vi "App - analyze RUS V6.vi"() -> ()   [LabVIEW 2015] (continued)
  out "frequency points":dbl[](array[numeric])=[0.0, 0.0, 0.0, 0.0, 0.0, 0.0, 0.0, 0.0, 0.0, 0.0, 0.0, 0.0, 0.0, 0.0, 0.0, 0.0, 0.0, 0.0, 0.0, 0.0, 0.0, 0.0, 0.0, 0.0, 0.0, 0.0, 0.0, 0.0, 0.0, 0.0, 0.0, 0.0, 0.0, 0.0, 0.0, 0.0, 0.0, 0.0, 0.0, 0.0, 0.0, 0.0, 0.0, 0.0, 0.0, 0.0, 0.0, 0.0, 664.2436695290903, 664.2619309392137, 664.2805728990513, 664.2981443004336, 664.3188476258067, 664.3335964907527, 664.3536063641833, 664.3711441248129, 664.3886135894766, 664.4069577109009, 664.4245585272355, 664.4414683185125, 664.4601452577426, 664.4796852677678, 664.4980076667935, 664.5154310442224, 664.5338643964093, 664.5517885931691, 664.5704803534437, 664.588180324614, 664.6064246538435, 664.6239877084581, 664.6422601490035, 664.6602601074228, 664.6782562264044, 664.6963935252326, 664.7147754224831, 664.7329875150317, 664.7514539650158, 664.7696405311139, 664.7884789608521, 664.8081200534322, 664.8281506310057, 664.8464656256355, 664.8647360420077, 664.8826826665108, 664.9021630370361, 664.9200138534414, 664.9394190348338, 664.9570161356205, 664.9751037863994, 664.9946492766225, 665.013363493181, 665.0319666327775, 665.0514303799941, 665.070428839104, 665.0899681894765, 665.1092165846538, 665.128636002681, 665.1480453032892, 665.1669866582076, 665.185992115189, 665.2049981978538, 665.2252219651873, 665.2450117111404, 665.2636719185228, 665.2820790020305, 665.302621721353, 665.3209060628186, 665.3411726525135, 665.3602455630045, 665.3791825777425, 665.3983648536116, 665.4185749812924, 665.4389184365867, 665.4576110068883, 665.4746111668128, 665.4943966614766, 665.5130010905406, 665.532316198093, 665.5532332931765, 665.57156331953, 665.592509513559, 665.6111561314502, 665.6307876831706, 665.6495981705524, 665.6676827317286, 665.6875855513655, 665.7073536709393, 665.7270146903713, 665.7475776559688, 665.7667570785509, 665.7853656920117, 665.8055568664535, 665.8247976415821, 665.8450275889691, 665.8652215366186, 665.8855803249663, 665.9069182376624, 665.9269377443005, 665.9465552746622, 665.9681031960093, 665.9882719429886, 666.0103637387408, 666.0300130208008, 666.0483020662261, 666.067358184188, 666.0861004254415, 666.1047052834762, 666.12482136998, 666.140704057652, 666.1610854922133, 666.1802100253361, 666.2003193033272, 666.2201606193609, 666.23899502151, 666.257459442358, 666.2778888148354, 666.2970981562802, 666.3156869001568, 666.3357577270784, 666.3558831541329, 666.3762094650621, 666.3976643168794, 666.4187151485258, 666.4383021086978, 666.4551854285005, 666.4720190334131, 666.4896912216159, 666.5084730527226, 666.5273905158227, 666.5408565163474, 666.5638551761065, 666.584524931986, 666.5994517164672, 666.6209744644639, 666.6398754592545, 666.6584173096262, 666.6738278296584, 666.692959166971, 666.7084573649482, 666.7295180919369, 666.7478022514588, 666.7684075589387, 666.7892001669214, 666.8168017277993, 666.8378173116613, 666.8546119137043, 666.8518486216516, 666.8670899449811, 666.8864924413293, 666.9049225640731, 666.9154225888688, 666.9360592058572, 666.9893085918818, 667.023179450894, 667.0181290997397, 667.0522165263105, 667.0670953246381, 667.0830991408355, 667.0958987277553, 667.1178151875246, 667.1376282461717, 667.1555761001051, 667.1729816030107, 667.1877067469779, 667.2026820856647, 667.2204079387552, 667.2371268200717, 667.2364415496808, 667.2762898680271, 667.2972094216088, 667.3167356990505, 667.3324754640709, 667.3490257970444, 667.3649515647236, 667.3831987020516, 667.3988052282629, 667.4131682428546, 667.4308567999159, 667.4487531200956, 667.4658300241209, 667.4848884179092, 667.5023892207363, 667.5167865078748, 667.530667219577, 667.5446936387285, 667.5507361439306, 667.5713768371177, 667.5871571554018, 667.603372353538, 667.6196504795548, 667.6345004307237, 667.6414584582035, 667.6596980423662, 667.6762506062214, 667.6919916866713, 667.704330610667, 667.7178274337781, 667.7315679125422, 667.7469406174972, 667.7605274396784, 667.772514287168, 667.7857246989796, 667.7975632145829, 667.8113824108048, 667.8259629307869, 667.8339870162451, 667.846314585591, 667.8533606686503, 667.8697794122957, 667.8814288240087, 667.8943565204472, 667.9070637171257, 667.9189901657315, 667.9290708716037, 667.9412342117888, 667.9478689614617, 667.9595344300756, 667.9715429031386, 667.98053690319, 667.9933159378816, 668.0042574571033, 668.0186275854775, 668.0261021371313, 668.038205785295, 668.0502969770072, 668.0581032164006, 668.0629833326522, 668.0682070709669, 668.0806358264088, 668.0819765634108, 668.0941556665481, 668.1086689007784, 668.1154417247612, 668.1232509827006, 668.1252877234232, 668.1324581018087, 668.1449136803938, 668.1500479338042, 668.1552952835116, 668.1649667431813, 668.1727890439503, 668.1779102230967, 668.1880252548099, 668.192804963829, 668.2024272814265, 668.2077960895239, 668.216668111389, 668.2220891882298, 668.2279899714331, 668.2341074013727, 668.2403250081744, 668.2467222103966, 668.2497252249998, 668.2550593154574, 668.2609151074342, 668.2619254491482, 668.270115071191, 668.276245083583, 668.2795802722522, 668.2870233031718, 668.2869168107318, 668.2934784041765, 668.3008315870534, 668.3028814309054, 668.3062964998082, 668.3103990781085, 668.310674127471, 668.3160212015783, 668.3205621538442, 668.3261810591241, 668.3339307703254, 668.3324079597492, 668.3322615543187, 668.3288000801537, 668.3337947654519, 668.3393724178951, 668.3408415336296, 668.3350781624661, 668.341978511539, 668.3443633787955, 668.3397547361191, 668.338634717693, 668.3411059711797, 668.3387712789065, 668.3427557708224, 668.3438270287197, 668.3463481103089, 668.3455084349229, 668.3450708618282, 668.3433267141062, 668.3444873126522, 668.3461478794261, 668.3457969116931, 668.3464465453555, 668.3409387012916, 668.3392344820684, 668.3394447248988, 668.3369686011712, 668.3366293662327, 668.3323623372692, 668.3318352391343, 668.3346922322422, 668.3330864941908, 668.3219517274852, 668.3129997886653, 668.3140680165973, 668.3088794677242, 668.3109415026871, 668.3052156629583, 668.3064621156966, 668.2991530946135, 668.296337187602, 668.2941712628873, 668.2879323748828, 668.2827006729923, 668.2752935986506, 668.2706731525243, 668.265311084802, 668.2583083453824, 668.2568309954227, 668.251544958297, 668.2453085062731, 668.2394743021457, 668.2322266809226, 668.2226032955875, 668.2221912502285, 668.2178106776172, 668.2137975862624, 668.2079346540519, 668.2000760755379, 668.194062828963, 668.1891261636409, 668.1800061469135, 668.1744243080439, 668.167621356464, 668.1637736220466, 668.1572968562582, 668.1537550879266, 668.1449838049871, 668.135169475204, 668.1246913482574, 668.121193286822, 668.1101664128744, 668.0998885496297, 668.0911411970284, 668.0843412935199, 668.074848351984, 668.0672099835513, 668.0546726344026, 668.0432151630731, 668.0317886551247, 668.0206931728633, 668.0108019958866, 668.000884305955, 667.994986941211, 667.9845360403064, 667.9709114890906, 667.963154410693, 667.9559671880407, 667.9461007473978, 667.9364915226823, 667.9270848813279, 667.9206130476543, 667.9097751474013, 667.9032383407135, 667.900021351503, 667.8939948673919, 667.8857574673999, 667.8761489000353, 667.873197176711, 667.8687353967621, 667.8714445455947, 667.8742869887905, 667.8871818169091, 667.8929742135593, 667.8950769727215, 667.9087317249022, 667.9127020137031, 667.9290862382628, 667.9424835071507, 667.9529480751149, 667.9649600314765, 667.9769292525697, 667.9949531202576, 668.0129403654028, 668.0268805358065, 668.0419170256847, 668.0495978156077, 668.0649496135221, 668.0806226434124, 668.0882919601835, 668.0896160369514, 668.0963848127388, 668.0981322511478, 668.106726291208, 668.1148687330386, 668.1099013064036, 668.1117303235795, 668.1110147726321, 668.1116377961806, 668.1101255100197, 668.1053232498274, 668.1031913806788, 668.1004691432302, 668.0992433152304, 668.1003509236078, 668.1064053025405, 668.1052302227044, 668.1022726722371, 668.1004679566593, 668.0972424835554, 668.0965315443399, 668.0939847231178, 668.0907103744488, 668.0884812262261, 668.0853168502122, 668.0833849424677, 668.0812319431826, 668.076925264809, 668.0728404783213, 668.0649075247303, 668.0660057593828, 668.0603228410023, 668.0526848700105, 668.0459870419369, 668.0382438056512, 668.0317727144501, 668.0229320244955, 668.0104558389754, 668.0013835956787, 667.9844280868045, 667.9730328624377, 667.9597690228534, 667.9520044016398, 667.9421204350114, 667.9314512587483, 667.9245739426502, 667.915672183135, 667.9042185316268, 667.8931568087993, 667.8785430669695, 667.867203293899, 667.8547807071961, 667.8418460648647, 667.8284078259741, 667.8174456972619, 667.8098934060879, 667.7999931838958, 667.7879029943412, 667.7767811952523, 667.766686685923, 667.7537699797824, 667.7441411520185, 667.7346507175026, 667.7218411788447, 667.7090832290504, 667.6987650095127, 667.6847550615028, 667.6716677581467, 667.6622092104991, 667.6494194591486, 667.6370796373111, 667.6271523663532, 667.616063077065, 667.5996159742031, 667.5849862740106, 667.5706432660058, 667.555832927336, 667.5428492141318, 667.5298004796668, 667.515440025869, 667.4995586436626, 667.4860922618307, 667.4736345533211, 667.4573357267553, 667.4424028954636, 667.4251980802276, 667.41000498982, 667.3944561053353, 667.3780759125216, 667.3663738953067, 667.3507898349178, 667.3338926093543, 667.3173685004768, 667.3005746288229, 667.2855690828252, 667.2692762902061, 667.2515590922309, 667.231376618077, 667.2146515753702, 667.1959425135124, 667.1780248365252, 667.1610973636662, 667.1361303785343, 667.1181117945565, 667.0987327287644, 667.0822028525415, 667.0647376572853, 667.0441866711889, 667.0271022203252, 667.0058178404381, 666.9844113515632, 666.9627164169844, 666.9433323926924, 666.9265821241922, 666.9065573278365, 666.8876756545675, 666.8690344911956, 666.8501315259728, 666.8344740108262, 666.8133340701726, 666.7935666574476, 666.7737931328093, 666.7536060450417, 666.7360341780229, 666.714098457095, 666.6950355612224, 666.675358388109, 666.6563167311539, 666.6383957613137, 666.6180927901069, 666.6002578587484, 666.581167167379, 666.5603597826648, 666.5413006512346, 666.5227729307114, 666.5025407776955, 666.4839616406631, 666.4635687138494, 666.4427909660764, 666.4214629416866, 666.4027073662497, 666.3832582108636, 666.3597242998917, 666.3423861780827, 666.3219837699494, 666.3027074087813, 666.2832044829721, 666.2547956648915, 666.2349515696993, 666.2143601194327, 666.1961380017648, 666.1741792701555, 666.1532060539795, 666.134360050069, 666.1144609518154, 666.0941688470095, 666.0718120080683, 666.0514464195873, 666.0325514837056, 666.009795226544, 665.9953474434808, 665.9751947106768, 665.9553477881376, 665.9343195300057, 665.9126957276022, 665.893856538965, 665.8735587517352, 665.8525097864081, 665.8348091435408, 665.8124994707074, 665.7921823307441, 665.770336097026, 665.751169981811, 665.7310500779857, 665.7095388817693, 665.6890167901994, 665.666392459161, 665.6483705534005, 665.6281709996543, 665.6073287703097, 665.5905919172243, 665.5700736081353, 665.5494957126687, 665.5288680893714, 665.5099899305785, 665.4902430620257, 665.4692472952553, 665.4499677322567, 665.4301516983661, 0.0, 0.0, 0.0, 665.3000947405819, 665.2801278621953, 665.2619142461758, 665.2441266774955, 665.2240080628333, 665.2045077919724, 665.183555272565, 665.170171669107, 665.1523314137073, 665.1325777519697, 665.1126173659541, 665.0915026087613, 665.0706732652532, 665.054034449722, 665.0338682665438, 665.0132269511125, 664.9933134080237, 664.9763291448037, 664.9564180576857, 664.9357800881095, 664.9153463888829, 664.8962985459169, 664.877249248592, 664.8577998829521, 664.8386786299899, 664.8188133493377, 664.8002015323394, 664.7795151476013, 664.7593151593608, 664.7400281342468, 664.7196311232841, 664.7007475651434, 664.6803637054721, 664.6597602636057, 664.6404420947947, 664.6201051910199, 664.5980460508742, 664.5800253851179, 664.5603925639282, 664.5418250189807, 664.5225693944557, 664.5035369558955, 664.4828049621776, 664.465505288, 664.4465122323005, 664.4269581428752, 664.4071198861543, 664.3873432834985, 664.3683940302727, 664.3480022893341, 664.3290848387534, 664.3099632939094, 664.2898717746746, 664.2707763707501, 664.2525985561252, 664.2332987241489, 664.2145643903633, 664.1958790605045, 664.17627848522, 664.1574446299836, 664.1383117517026, 664.1189516478559, 664.0996935583665, 664.0810745610588, 664.0621135285246, 664.0435393826916, 664.0255098851464, 664.0073679349201, 663.9886506388516, 663.9687076319055, 663.9499123640444, 663.9300692915438, 663.9104025268014, 663.8919973297286, 663.8725802754554, 663.8531342977661, 663.834753319743, 663.8174664217973, 663.7976768196731, 663.7786903386511, 663.7592398477731, 663.738826060015, 663.7213392465111, 663.7025470782887, 663.6810373710007, 663.6638983583827, 663.6439303978735, 663.6241437684071, 663.6053258833265, 663.5880613487568, 663.5698546355719, 663.5515429002106, 663.5338391109882, 663.5159545204048, 663.4970989685446, 663.4769127694987, 663.4981912028674, 663.499400259395, 663.450380905746, 663.468044758759, 663.4473219222272, 663.321849078867, 0.0, 663.321849078867, 0.0, 0.0, 0.0, 0.0, 0.0, 0.0, 663.2012958301423, 0.0, 663.1800332004171, 663.1586234942882, 0.0, 663.1389266485459, 0.0, 663.1015876451874, 0.0, 663.0600120819944, 0.0, 663.0228973120825, 0.0, 662.9654599727345, 662.9654599727345, 0.0, 0.0, 0.0, 0.0, 0.0, 0.0, 0.0, 0.0, 0.0, 0.0, 0.0, 0.0, 0.0, 0.0, 0.0, 0.0, 0.0, 0.0, 0.0, 0.0, 0.0, 0.0, 0.0, 0.0, 0.0, 0.0, 0.0, 0.0, 0.0, 0.0, 0.0, 0.0, 0.0, 0.0, 0.0, 0.0, 0.0, 0.0, 0.0, 0.0, 0.0, 0.0, 0.0, 0.0, 0.0, 0.0, 0.0, 0.0, 0.0, 0.0, 0.0, 0.0, 0.0, 0.0, 0.0, 0.0, 0.0, 0.0, 0.0, 0.0, 0.0, 0.0, 0.0, 0.0, 0.0, 0.0, 0.0, 0.0, 0.0, 0.0, 0.0, 0.0, 0.0, 0.0, 0.0, 0.0, 0.0, 0.0, 0.0, 0.0, 0.0, 0.0, 0.0, 0.0, 0.0, 0.0, 0.0, 0.0, 0.0, 0.0, 0.0, 0.0, 0.0, 0.0, 0.0, 0.0, 0.0, 0.0, 0.0, 0.0, 0.0, 0.0, 0.0, 0.0, 0.0, 0.0, 0.0, 0.0, 0.0, 0.0, 0.0, 0.0, 0.0, 0.0, 0.0, 0.0, 0.0, 0.0, 0.0, 0.0, 0.0, 0.0, 0.0, 0.0, 0.0, 0.0, 0.0, 0.0, 0.0, 0.0, 0.0, 0.0, 0.0, 0.0, 0.0, 0.0, 0.0, 0.0, 0.0, 0.0, 0.0, 0.0, 0.0, 0.0, 0.0, 0.0, 0.0, 0.0, 0.0, 0.0, 0.0, 0.0, 0.0, 0.0, 0.0, 0.0, 0.0, 0.0, 0.0, 0.0, 0.0, 0.0, 0.0, 0.0, 0.0, 0.0, 0.0, 0.0, 0.0, 0.0, 0.0, 0.0, 0.0, 0.0, 0.0, 0.0, 0.0, 0.0, 0.0, 0.0, 0.0, 0.0, 0.0, 0.0, 0.0, 0.0, 0.0, 0.0, 0.0, 0.0, 0.0, 0.0, 0.0, 0.0, 0.0, 0.0, 0.0, 0.0, 0.0, 0.0, 0.0, 0.0, 0.0, 0.0, 0.0, 0.0, 0.0, 0.0, 0.0, 0.0, 0.0, 0.0, 0.0, 0.0, 0.0, 0.0, 0.0, 0.0, 0.0, 0.0, 0.0, 0.0, 0.0, 0.0, 0.0, 0.0, 0.0, 0.0, 0.0, 0.0, 0.0, 0.0, 0.0, 0.0, 0.0, 0.0, 0.0, 0.0, 0.0, 0.0, 0.0, 0.0, 0.0, 0.0, 0.0, 0.0, 0.0, 0.0, 0.0, 0.0, 0.0, 0.0, 0.0, 0.0, 0.0, 0.0, 0.0, 0.0, 0.0, 0.0, 0.0, 0.0, 0.0, 0.0, 0.0, 0.0, 0.0, 0.0, 0.0, 0.0, 0.0, 0.0, 0.0, 0.0, 0.0, 0.0, 0.0, 0.0, 0.0, 0.0, 0.0, 0.0, 0.0, 0.0, 0.0, 0.0, 0.0, 0.0, 0.0, 0.0, 0.0, 0.0, 0.0, 0.0, 0.0, 0.0, 0.0, 0.0, 0.0, 0.0, 0.0, 0.0, 0.0, 0.0, 0.0, 0.0, 0.0, 0.0, 0.0, 0.0, 0.0, 0.0, 0.0, 0.0, 0.0, 0.0, 0.0, 0.0, 0.0, 0.0, 0.0, 0.0, 0.0, 0.0, 0.0, 0.0, 0.0, 0.0, 0.0, 0.0, 0.0, 0.0, 0.0, 0.0, 0.0, 0.0, 0.0, 0.0, 0.0, 0.0, 0.0, 0.0, 0.0, 0.0, 0.0, 0.0, 0.0, 0.0, 0.0, 0.0, 0.0, 0.0, 0.0, 0.0, 0.0, 0.0, 0.0, 0.0, 0.0, 0.0, 0.0, 0.0, 0.0, 0.0, 0.0, 0.0, 0.0, 0.0, 0.0, 0.0, 0.0, 0.0, 0.0, 0.0, 0.0, 0.0, 0.0, 0.0, 0.0, 0.0, 0.0, 0.0, 0.0, 0.0, 0.0, 0.0, 0.0, 0.0, 0.0, 0.0, 0.0, 0.0, 0.0, 0.0, 0.0, 0.0, 0.0, 0.0, 0.0, 0.0, 0.0, 0.0, 0.0, 0.0, 0.0, 0.0, 0.0, 0.0, 0.0, 0.0, 0.0, 0.0, 0.0, 0.0, 0.0, 0.0, 0.0, 0.0, 0.0, 0.0, 0.0, 0.0, 0.0, 0.0, 0.0, 0.0, 0.0, 0.0, 0.0, 0.0, 0.0, 0.0, 0.0, 0.0, 0.0, 0.0, 0.0, 0.0, 0.0, 0.0, 0.0, 0.0, 0.0, 0.0, 0.0, 0.0, 0.0, 0.0, 0.0, 0.0, 0.0, 0.0, 0.0, 0.0, 0.0, 0.0, 0.0, 0.0, 0.0, 0.0, 0.0, 0.0, 0.0, 0.0, 0.0, 0.0, 0.0, 0.0, 0.0, 0.0, 0.0, 0.0, 0.0, 0.0, 0.0, 0.0, 0.0, 0.0, 0.0, 0.0, 0.0, 0.0, 0.0, 0.0, 0.0, 0.0, 0.0, 0.0, 0.0, 0.0, 0.0, 0.0, 0.0, 0.0, 0.0, 0.0, 0.0, 0.0, 0.0, 0.0, 0.0, 0.0, 0.0, 0.0, 0.0, 0.0, 0.0, 0.0, 0.0, 0.0, 0.0, 0.0, 0.0, 0.0, 0.0, 0.0, 0.0, 0.0, 0.0, 0.0, 0.0, 0.0, 0.0, 0.0, 0.0, 0.0, 0.0, 0.0, 0.0, 0.0, 0.0, 0.0, 0.0, 0.0, 0.0, 0.0, 0.0, 0.0, 0.0, 0.0, 0.0, 0.0, 0.0, 0.0, 0.0, 0.0, 0.0, 0.0, 0.0, 0.0, 0.0, 0.0, 0.0, 0.0, 0.0, 0.0, 0.0, 0.0, 0.0, 0.0, 0.0, 0.0, 0.0, 0.0, 0.0, 0.0, 0.0, 0.0, 0.0, 0.0, 0.0, 0.0, 0.0, 0.0, 0.0, 0.0, 0.0, 0.0, 0.0, 0.0, 0.0, 0.0, 0.0, 0.0, 0.0, 0.0, 0.0, 0.0, 0.0, 0.0, 0.0, 0.0, 0.0, 0.0, 0.0, 0.0, 0.0, 0.0, 0.0, 0.0, 0.0, 0.0, 0.0, 0.0, 0.0, 0.0, 0.0, 0.0, 0.0, 0.0, 0.0, 0.0, 0.0, 0.0, 0.0, 0.0, 0.0, 0.0, 0.0, 0.0, 0.0, 0.0, 0.0, 0.0, 0.0, 0.0, 0.0, 0.0, 0.0, 0.0, 0.0, 0.0, 0.0, 0.0, 0.0, 0.0, 0.0, 0.0, 0.0, 0.0, 0.0, 0.0, 0.0, 0.0, 0.0, 0.0, 0.0, 0.0, 0.0, 0.0, 0.0, 0.0, 0.0, 0.0, 0.0, 0.0, 0.0, 0.0, 0.0, 0.0, 0.0, 0.0, 0.0, 0.0, 0.0, 0.0, 0.0, 0.0, 0.0, 0.0, 0.0, 0.0, 0.0, 0.0, 0.0, 0.0, 0.0, 0.0, 0.0, 0.0, 0.0, 0.0, 0.0, 0.0, 0.0, 0.0, 0.0, 0.0, 0.0, 0.0, 0.0, 0.0, 0.0, 0.0, 0.0, 0.0, 0.0, 0.0, 0.0, 0.0, 0.0, 0.0, 0.0, 0.0, 0.0, 0.0, 0.0, 0.0, 0.0, 0.0, 0.0, 0.0, 0.0, 0.0, 0.0, 0.0, 0.0, 0.0, 0.0, 0.0, 0.0, 0.0, 0.0, 0.0, 0.0, 0.0, 0.0, 0.0, 0.0, 0.0, 0.0, 0.0, 0.0, 0.0, 0.0, 0.0, 0.0, 0.0, 0.0, 0.0, 0.0, 0.0, 0.0, 0.0, 0.0, 0.0, 0.0, 0.0, 0.0, 0.0, 0.0, 0.0, 0.0, 0.0, 0.0, 0.0, 0.0, 0.0, 0.0, 0.0, 0.0, 0.0, 0.0, 0.0, 0.0, 0.0, 0.0, 0.0, 0.0, 0.0, 0.0, 0.0, 0.0, 0.0, 0.0, 0.0, 0.0, 0.0, 0.0, 0.0, 0.0, 0.0, 0.0, 0.0, 0.0, 0.0, 0.0, 0.0, 0.0, 0.0, 0.0, 0.0, 0.0, 0.0, 0.0, 0.0, 0.0, 0.0, 0.0, 0.0, 0.0, 0.0, 0.0, 0.0, 0.0, 0.0, 0.0, 0.0, 0.0, 0.0, 0.0, 0.0, 0.0, 0.0, 0.0, 0.0, 0.0, 0.0, 0.0, 0.0, 0.0, 0.0, 0.0, 0.0, 0.0, 0.0, 0.0, 0.0, 0.0, 0.0, 0.0, 0.0, 0.0, 0.0, 0.0, 0.0, 0.0, 0.0, 0.0, 0.0, 0.0, 0.0, 0.0, 0.0, 0.0, 0.0, 0.0, 0.0, 0.0, 0.0, 0.0, 0.0, 0.0, 0.0, 0.0, 0.0, 0.0, 0.0, 0.0, 0.0, 0.0, 0.0, 0.0, 0.0, 0.0, 0.0, 0.0, 0.0, 0.0, 0.0, 0.0, 0.0, 0.0, 0.0, 0.0, 0.0, 0.0, 0.0, 0.0, 0.0, 0.0, 0.0, 0.0, 0.0, 0.0, 0.0, 0.0, 0.0, 0.0, 0.0, 0.0, 0.0, 0.0, 0.0, 0.0, 0.0, 0.0, 0.0, 0.0, 0.0, 0.0, 0.0, 0.0, 0.0, 0.0, 0.0, 0.0, 0.0, 0.0, 0.0, 0.0, 0.0, 0.0, 0.0, 0.0, 0.0, 0.0, 0.0, 0.0, 0.0, 0.0, 0.0, 0.0, 0.0, 0.0, 0.0, 0.0, 0.0, 0.0, 0.0, 0.0, 0.0, 0.0, 0.0, 0.0, 0.0, 0.0, 0.0, 0.0, 0.0, 0.0, 0.0, 0.0, 0.0, 0.0, 0.0, 0.0, 0.0, 0.0, 0.0, 0.0, 0.0, 0.0, 0.0, 0.0, 0.0, 0.0, 0.0, 0.0, 0.0, 0.0, 0.0, 0.0, 0.0, 0.0, 0.0, 0.0, 0.0, 0.0, 0.0, 0.0, 0.0, 0.0, 0.0, 0.0, 0.0, 0.0, 0.0, 0.0, 0.0, 0.0, 0.0, 0.0, 0.0, 0.0, 0.0, 0.0, 0.0, 0.0, 0.0, 0.0, 0.0, 0.0, 0.0, 0.0, 0.0, 0.0, 0.0, 0.0, 0.0, 0.0, 0.0, 0.0, 0.0, 0.0, 0.0, 0.0, 0.0, 0.0, 0.0, 0.0, 0.0, 0.0, 0.0, 0.0, 0.0, 0.0, 0.0, 0.0, 0.0, 0.0, 0.0, 0.0, 0.0, 0.0, 0.0, 0.0, 0.0, 0.0, 0.0, 0.0, 0.0, 0.0, 0.0, 0.0, 0.0, 0.0, 0.0, 0.0, 0.0, 0.0, 0.0, 0.0, 0.0, 0.0, 0.0, 0.0, 0.0, 0.0, 0.0, 0.0, 0.0, 0.0, 0.0, 0.0, 0.0, 0.0, 0.0, 0.0, 0.0, 0.0, 0.0, 0.0, 0.0, 0.0, 0.0, 0.0, 0.0, 0.0, 0.0, 0.0, 0.0, 0.0, 0.0, 0.0, 0.0, 0.0, 0.0, 0.0, 0.0, 0.0, 0.0, 0.0, 0.0, 0.0, 0.0, 0.0, 0.0, 0.0, 0.0, 0.0, 0.0, 0.0, 0.0, 0.0, 0.0, 0.0, 0.0, 0.0, 0.0, 0.0, 0.0, 0.0, 0.0, 0.0, 0.0, 0.0, 0.0, 0.0, 0.0, 0.0, 0.0, 0.0, 0.0, 0.0, 0.0, 0.0, 0.0, 0.0, 0.0, 0.0, 0.0, 0.0, 0.0, 0.0, 0.0, 0.0, 0.0, 0.0, 0.0, 0.0, 0.0, 0.0, 0.0, 0.0, 0.0, 0.0, 0.0, 0.0, 0.0, 0.0, 0.0, 0.0, 0.0, 0.0, 0.0, 0.0, 0.0, 0.0, 0.0, 0.0, 0.0, 0.0, 0.0, 0.0, 0.0, 0.0, 0.0, 0.0, 0.0, 0.0, 0.0, 0.0, 0.0, 0.0, 0.0, 0.0, 0.0, 0.0, 0.0, 0.0, 0.0, 0.0, 0.0, 0.0, 0.0, 0.0, 0.0, 0.0, 0.0, 0.0, 0.0, 0.0, 0.0, 0.0, 0.0, 0.0, 0.0, 0.0, 0.0, 0.0, 0.0, 0.0, 0.0, 0.0, 0.0, 0.0, 0.0, 0.0, 0.0, 0.0, 0.0, 0.0, 0.0, 0.0, 0.0, 0.0, 0.0, 0.0, 0.0, 0.0, 0.0, 0.0, 0.0, 0.0, 0.0, 0.0, 0.0, 0.0, 0.0, 0.0, 0.0, 0.0, 0.0, 0.0, 0.0, 0.0, 0.0, 0.0, 0.0, 0.0, 0.0, 0.0, 0.0, 0.0, 0.0, 0.0, 0.0, 0.0, 0.0, 0.0, 0.0, 0.0, 0.0, 0.0, 0.0, 0.0, 0.0, 0.0, 0.0, 0.0, 0.0, 0.0, 0.0, 0.0, 0.0, 0.0, 0.0, 0.0, 0.0, 0.0, 0.0, 0.0, 0.0, 0.0, 0.0, 0.0, 0.0, 0.0, 0.0, 0.0, 0.0, 0.0, 0.0, 0.0, 0.0, 0.0, 0.0, 0.0, 0.0, 0.0, 0.0, 0.0, 0.0, 0.0, 0.0, 0.0, 0.0, 0.0, 0.0, 0.0, 0.0, 0.0, 0.0, 0.0, 0.0, 0.0, 0.0, 0.0, 0.0, 0.0, 0.0, 0.0, 0.0, 0.0, 0.0, 0.0, 0.0, 0.0, 0.0, 0.0, 0.0, 0.0, 0.0, 0.0, 0.0, 0.0, 0.0, 0.0, 0.0, 0.0, 0.0, 0.0, 0.0, 0.0, 0.0, 0.0, 0.0, 0.0, 0.0, 0.0, 0.0, 0.0, 0.0, 0.0, 0.0, 0.0, 0.0, 0.0, 0.0, 0.0, 0.0, 0.0, 0.0, 0.0, 0.0, 0.0, 0.0, 0.0, 0.0, 0.0, 0.0, 0.0, 0.0, 0.0, 0.0, 0.0, 0.0, 0.0, 0.0, 0.0, 0.0, 0.0, 0.0, 0.0, 0.0, 0.0, 0.0, 0.0, 0.0, 0.0, 0.0, 0.0, 0.0, 0.0, 0.0, 0.0, 0.0, 0.0, 0.0, 0.0, 0.0, 0.0, 0.0, 0.0, 0.0, 0.0, 0.0, 0.0, 0.0, 0.0, 0.0, 0.0, 0.0, 0.0, 0.0, 0.0, 0.0, 0.0, 0.0, 0.0, 0.0, 0.0, 0.0, 0.0, 0.0, 0.0, 0.0]
  out "all:max omega":dbl=2551.395387007042
  out "all:min omega":dbl=501.5
  out "format version":string="A1"
  out "delta-f points":dbl[](array[numeric])=[nan, nan, nan, nan, nan, nan, nan, nan, nan, nan, nan, nan, nan, nan, nan, nan, nan, nan, nan, nan, nan, nan, nan, nan, nan, nan, nan, nan, nan, nan, nan, nan, nan, nan, nan, nan, nan, nan, nan, nan, nan, nan, nan, nan, nan, nan, nan, nan, nan, nan, nan, nan, nan, nan, nan, nan, nan, nan, nan, nan, nan, nan, nan, nan, nan, nan, nan, nan, nan, nan, nan, nan, nan, nan, nan, nan, nan, nan, nan, nan, nan, nan, nan, nan, nan, nan, nan, nan, nan, nan, nan, nan, nan, nan, nan, nan, nan, nan, nan, nan, nan, nan, nan, nan, nan, nan, nan, nan, nan, nan, nan, nan, nan, nan, nan, nan, nan, nan, nan, nan, nan, nan, nan, nan, nan, nan, nan, nan, nan, nan, nan, nan, nan, nan, nan, nan, nan, nan, nan, nan, nan, nan, nan, nan, nan, nan, nan, nan, nan, nan, nan, nan, nan, nan, nan, nan, nan, nan, nan, nan, nan, nan, nan, nan, nan, nan, nan, nan, nan, nan, nan, nan, nan, nan, nan, nan, nan, nan, nan, nan, nan, nan, nan, nan, nan, nan, nan, nan, nan, nan, nan, nan, nan, nan, nan, nan, nan, nan, nan, nan, nan, nan, nan, nan, nan, nan, nan, nan, nan, nan, nan, nan, nan, nan, nan, nan, nan, nan, nan, nan, nan, nan, nan, nan, nan, nan, nan, nan, nan, nan, nan, nan, nan, nan, nan, nan, nan, nan, nan, nan, nan, nan, nan, nan, nan, nan, nan, nan, nan, nan, nan, nan, nan, nan, nan, nan, nan, nan, nan, nan, nan, nan, nan, nan, nan, nan, nan, nan, nan, nan, nan, nan, nan, nan, nan, nan, nan, nan, nan, nan, nan, nan, nan, nan, nan, nan, nan, nan, nan, nan, nan, nan, nan, nan, nan, nan, nan, nan, nan, nan, nan, nan, nan, nan, nan, nan, nan, nan, nan, nan, nan, nan, nan, nan, nan, nan, nan, nan, nan, nan, nan, nan, nan, nan, nan, nan, nan, nan, nan, nan, nan, nan, nan, nan, nan, nan, nan, nan, nan, nan, nan, nan, nan, nan, nan, nan, nan, nan, nan, nan, nan, nan, nan, nan, nan, nan, nan, nan, nan, nan, nan, nan, nan, nan, nan, nan, nan, nan, nan, nan, nan, nan, nan, nan, nan, nan, nan, nan, nan, nan, nan, nan, nan, nan, nan, nan, nan, nan, nan, nan, nan, nan, nan, nan, nan, nan, nan, nan, nan, nan, nan, nan, nan, nan, nan, nan, nan, nan, nan, nan, nan, nan, nan, nan, nan, nan, nan, nan, nan, nan, nan, nan, nan, nan, nan, nan, nan, nan, nan, nan, nan, nan, nan, nan, nan, nan, nan, nan, nan, nan, nan, nan, nan, nan, nan, nan, nan, nan, nan, nan, nan, nan, nan, nan, nan, nan, nan, nan, nan, nan, nan, nan, nan, nan, nan, nan, nan, nan, nan, nan, nan, nan, nan, nan, nan, nan, nan, nan, nan, nan, nan, nan, nan, nan, nan, nan, nan, nan, nan, nan, nan, nan, nan, nan, nan, nan, nan, nan, nan, nan, nan, nan, nan, nan, nan, nan, nan, nan, nan, nan, nan, nan, nan, nan, nan, nan, nan, nan, nan, nan, nan, nan, nan, nan, nan, nan, nan, nan, nan, nan, nan, nan, nan, nan, nan, nan, nan, nan, nan, nan, nan, nan, nan, nan, nan, nan, nan, nan, nan, nan, nan, nan, nan, nan, nan, nan, nan, nan, nan, nan, nan, nan, nan, nan, nan, nan, nan, nan, nan, nan, nan, nan, nan, nan, nan, nan, nan, nan, nan, nan, nan, nan, nan, nan, nan, nan, nan, nan, nan, nan, nan, nan, nan, nan, nan, nan, nan, nan, nan, nan, nan, nan, nan, nan, nan, nan, nan, nan, nan, nan, nan, nan, nan, nan, nan, nan, nan, nan, nan, nan, nan, nan, nan, nan, nan, nan, nan, nan, nan, nan, nan, nan, nan, nan, nan, nan, nan, nan, nan, nan, nan, nan, nan, nan, nan, nan, nan, nan, nan, nan, nan, nan, nan, nan, nan, nan, nan, nan, nan, nan, nan, nan, nan, nan, nan, nan, nan, nan, nan, nan, nan, nan, nan, nan, nan, nan, nan, nan, nan, nan, nan, nan, nan, nan, nan, nan, nan, nan, nan, nan, nan, nan, nan, nan, nan, nan, nan, nan, nan, nan, nan, nan, nan, nan, nan, nan, nan, nan, nan, nan, nan, nan, nan, nan, nan, nan, nan, nan, nan, nan, nan, nan, nan, nan, nan, nan, nan, nan, nan, nan, nan, nan, nan, nan, nan, nan, nan, nan, nan, nan, nan, nan, nan, nan, nan, nan, nan, nan, nan, nan, nan, nan, nan, nan, nan, nan, nan, nan, nan, nan, nan, nan, nan, nan, nan, nan, nan, nan, nan, nan, nan, nan, nan, nan, nan, nan, nan, nan, nan, nan, nan, nan, nan, nan, nan, nan, nan, nan, nan, nan, nan, nan, nan, nan, nan, nan, nan, nan, nan, nan, nan, nan, nan, nan, nan, nan, nan, nan, nan, nan, nan, nan, nan, nan, nan, nan, nan, nan, nan, nan, nan, nan, nan, nan, nan, nan, nan, nan, nan, nan, nan, nan, nan, nan, nan, nan, nan, nan, nan, nan, nan, nan, nan, nan, nan, nan, nan, nan, nan, nan, nan, nan, nan, nan, nan, nan, nan, nan, nan, nan, nan, nan, nan, nan, nan, nan, nan, nan, nan, nan, nan, nan, nan, nan, nan, nan, nan, nan, nan, nan, nan, nan, nan, nan, nan, nan, nan, nan, nan, nan, nan, nan, nan, nan, nan, nan, nan, nan, nan, nan, nan, nan, nan, nan, nan, nan, nan, nan, nan, nan, nan, nan, nan, nan, nan, nan, nan, nan, nan, nan, nan, nan, nan, nan, nan, nan, nan, nan, nan, nan, nan, nan, nan, nan, nan, nan, nan, nan, nan, nan, nan, nan, nan, nan, nan, nan, nan, nan, nan, nan, nan, nan, nan, nan, nan, nan, nan, nan, nan, nan, nan, nan, nan, nan, nan, nan, nan, nan, nan, nan, nan, nan, nan, nan, nan, nan, nan, nan, nan, nan, nan, nan, nan, nan, nan, nan, nan, nan, nan, nan, nan, nan, nan, nan, nan, nan, nan, nan, nan, nan, nan, nan, nan, nan, nan, nan, nan, nan, nan, nan, nan, nan, nan, nan, nan, nan, nan, nan, nan, nan, nan, nan, nan, nan, nan, nan, nan, nan, nan, nan, nan, nan, nan, nan, nan, nan, nan, nan, nan, nan, nan, nan, nan, nan, nan, nan, nan, nan, nan, nan, nan, nan, nan, nan, nan, nan, nan, nan, nan, nan, nan, nan, nan, nan, nan, nan, nan, nan, nan, nan, nan, nan, nan, nan, nan, nan, nan, nan, nan, nan, nan, nan, nan, nan, nan, nan, nan, nan, nan, nan, nan, nan, nan, nan, nan, nan, nan, nan, nan, nan, nan, nan, nan, nan, nan, nan, nan, nan, nan, nan, nan, nan, nan, nan, nan, nan, nan, nan, nan, nan, nan, nan, nan, nan, nan, nan, nan, nan, nan, nan, nan, nan, nan, nan, nan, nan, nan, nan, nan, nan, nan, nan, nan, nan, nan, nan, nan, nan, nan, nan, nan, nan, nan, nan, nan, nan, nan, nan, nan, nan, nan, nan, nan, nan, nan, nan, nan, nan, nan, nan, nan, nan, nan, nan, nan, nan, nan, nan, nan, nan, nan, nan, nan, nan, nan, nan, nan, nan, nan, nan, nan, nan, nan, nan, nan, nan, nan, nan, nan, nan, nan, nan, nan, nan, nan, nan, nan, nan, nan, nan, nan, nan, nan, nan, nan, nan, nan, nan, nan, nan, nan, nan, nan, nan, nan, nan, nan, nan, nan, nan, nan, nan, nan, nan, nan, nan, nan, nan, nan, nan, nan, nan, nan, nan, nan, nan, nan, nan, nan, nan, nan, nan, nan, nan, nan, nan, nan, nan, nan, nan, nan, nan, nan, nan, nan, nan, nan, nan, nan, nan, nan, nan, nan, nan, nan, nan, nan, nan, nan, nan, nan, nan, nan, nan, nan, nan, nan, nan, nan, nan, nan, nan, nan, nan, nan, nan, nan, nan, nan, nan, nan, nan, nan, nan, nan, nan, nan, nan, nan, nan, nan, nan, nan, nan, nan, nan, nan, nan, nan, nan, nan, nan, nan, nan, nan, nan, nan, nan, nan, nan, nan, nan, nan, nan, nan, nan, nan, nan, nan, nan, nan, nan, nan, nan, nan, nan, nan, nan, nan, nan, nan, nan, nan, nan, nan, nan, nan, nan, nan, nan, nan, nan, nan, nan, nan, nan, nan, nan, nan, nan, nan, nan, nan, nan, nan, nan, nan, nan, nan, nan, nan, nan, nan, nan, nan, nan, nan, nan, nan, nan, nan, nan, nan, nan, nan, nan, nan, nan, nan, nan, nan, nan, nan, nan, nan, nan, nan, nan, nan, nan, nan, nan, nan, nan, nan, nan, nan, nan, nan, nan, nan, nan, nan, nan, nan, nan, nan, nan, nan, nan, nan, nan, nan, nan, nan, nan, nan, nan, nan, nan, nan, nan, nan, nan, nan, nan, nan, nan, nan, nan, nan, nan, nan, nan, nan, nan, nan, nan, nan, nan, nan, nan, nan, nan, nan, nan, nan, nan, nan, nan, nan, nan, nan, nan, nan, nan, nan, nan, nan, nan, nan, nan, nan, nan, nan, nan, nan, nan, nan, nan, nan, nan, nan, nan, nan, nan, nan, nan, nan, nan, nan, nan, nan, nan, nan, nan, nan, nan, nan, nan, nan, nan, nan, nan, nan, nan, nan, nan, nan, nan, nan, nan, nan, nan, nan, nan, nan, nan, nan, nan, nan, nan, nan, nan, nan, nan, nan, nan, nan, nan, nan, nan, nan, nan, nan, nan, nan, nan, nan, nan, nan, nan, nan, nan, nan, nan, nan, nan, nan, nan, nan, nan, nan, nan, nan, nan, nan, nan, nan, nan, nan, nan, nan, nan, nan, nan, nan, nan, nan, nan, nan, nan, nan, nan, nan, nan, nan, nan, nan, nan, nan, nan, nan, nan, nan, nan, nan, nan, nan, nan, nan, nan, nan, nan, nan, nan, nan, nan, nan, nan, nan, nan, nan, nan, nan, nan, nan, nan, nan, nan, nan, nan, nan, nan, nan, nan, nan, nan, nan, nan, nan, nan, nan, nan, nan, nan, nan, nan, nan, nan, nan, nan, nan, nan, nan, nan, nan, nan, nan, nan, nan, nan, nan, nan, nan, nan, nan, nan, nan, nan, nan, nan, nan, nan, nan, nan, nan, nan, nan, nan, nan, nan, nan, nan, nan, nan, nan, nan, nan, nan, nan, nan, nan, nan, nan, nan, nan, nan, nan, nan, nan, nan, nan, nan, nan, nan, nan, nan, nan, nan, nan, nan, nan, nan, nan, nan, nan, nan, nan, nan, nan, nan, nan, nan, nan, nan, nan, nan, nan, nan, nan, nan, nan, nan, nan, nan, nan, nan, nan, nan, nan, nan, nan, nan, nan, nan, nan, nan, nan, nan, nan, nan, nan, nan, nan, nan, nan, nan, nan, nan, nan, nan, nan, nan, nan, nan, nan, nan, nan, nan, nan, nan, nan, nan, nan, nan, nan, nan, nan, nan, nan, nan, nan, nan, nan, nan, nan, nan, nan, nan, nan, nan, nan, nan, nan, nan, nan, nan, nan, nan, nan, nan, nan, nan, nan, nan, nan, nan, nan, nan, nan, nan, nan, nan, nan, nan, nan, nan, nan, nan, nan, nan, nan, nan, nan, nan, nan, nan, nan, nan, nan, nan, nan, nan, nan, nan, nan, nan, nan, nan, nan, nan, nan, nan, nan, nan, nan, nan, nan, nan, nan, nan, nan, nan, nan, nan, nan, nan, nan, nan, nan, nan, nan, nan, nan, nan, nan, nan, nan, nan, nan, nan, nan, nan, nan, nan, nan, nan, nan, nan, nan, nan, nan, nan, nan, nan, nan, nan, nan, nan, nan, nan, nan, nan, nan, nan, nan, nan, nan, nan, nan, nan, nan, nan, nan, nan, nan, nan, nan, nan, nan, nan, nan, nan, nan, nan, nan, nan, nan, nan, nan, nan, nan, nan, nan, nan, nan, nan, nan, nan, nan, nan, nan, nan, nan, nan, nan, nan, nan, nan, nan, nan, nan, nan, nan, nan, nan, nan, nan, nan, nan, nan, nan, nan, nan, nan, nan, nan, nan, nan, nan, nan, nan, nan, nan, nan, nan, nan, nan, nan, nan, nan, nan, nan, nan, nan, nan, nan, nan, nan, nan, nan, nan, nan, nan, nan, nan, nan, nan, nan, nan, nan, nan, nan, nan, nan, nan, nan, nan, nan, nan, nan, nan, nan, nan, nan, nan, nan, nan, nan, nan, nan, nan, nan, nan, nan, nan, nan, nan, nan, nan, nan, nan, nan, nan, nan, nan, nan, nan, nan, nan, nan, nan, nan, nan, nan, nan, nan, nan, nan, nan, nan, nan, nan, nan, nan, nan, nan, nan, nan, nan, nan, nan, nan, nan, nan, nan, nan, nan, nan, nan, nan, nan, nan, nan, nan, nan, nan, nan, nan, nan, nan, nan, nan, nan, nan, nan, nan, nan, nan, nan, nan, nan, nan, nan, nan, nan, nan, nan, nan, nan, nan, nan, nan, nan, nan, nan, nan, nan, nan, nan, nan, nan, nan, nan, nan, nan, nan, nan, nan, nan, nan, nan, nan, nan, nan, nan, nan, nan, nan, nan, nan, nan, nan, nan, nan, nan, nan, nan, nan, nan, nan, nan, nan, nan, nan, nan, nan, nan, nan, nan, nan, nan, nan, nan, nan, nan, nan, nan, nan, nan, nan, nan, nan, nan, nan, nan, nan, nan, nan, nan, nan, nan, nan, nan, nan]
